vi "InitializeGUIControls.vi"(0 "Timing Plot":refnum<vi>, 1 "Save shot data":refnum<vi>, 2 "Discard shot data":refnum<vi>, 3 "Shot Quality":refnum<vi>, 4 "Fire Experiment":refnum<vi>, 5 "Abort":refnum<vi>) -> ()   [LabVIEW 2014]
doc: "Initialize various front panel GUI items. Such as reset the timing plot, disable the save/discard shot data buttons, etc."
uses:
  Controls/ShotQualityEnum.ctl
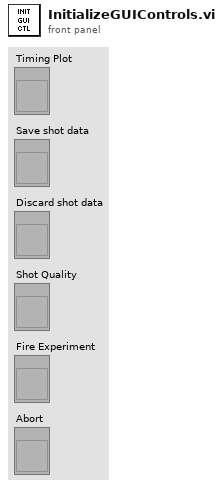
[diagram p1: front panel]
types:
  T1 = enum8{"Enabled", "Disabled", "Disabled and Grayed Out"}
  T2 = typedef "ShotQualityEnum.ctl" = enum32{"-2", "-1", "1", "2", "3", "0"}
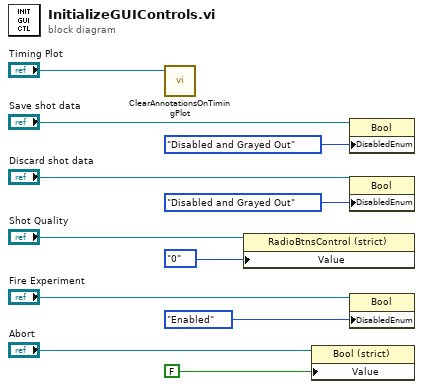
[diagram p0: block diagram]
diagram:
  n1 = call "ClearAnnotationsOnTimingPlot.vi"("Cluster in"="Timing Plot") -> ()  [unwired: 11 in]
  n2 = property class="RadioBtnsControl (strict)"(reference="Shot Quality", "Value"=ShotQualityEnum."0" ("Shot Quality")) -> ()  [unwired: 1 in, 2 out]
  n3 = property class="Bool (strict)"(reference="Abort", "Value"=FALSE) -> ()  [unwired: 1 in, 2 out]
  n4 = property class="Bool"(reference="Save shot data", "DisabledEnum"=T1."Disabled and Grayed Out" ("Disabled")) -> ()  [unwired: 1 in, 2 out]
  n5 = property class="Bool"(reference="Discard shot data", "DisabledEnum"=T1."Disabled and Grayed Out" ("Disabled")) -> ()  [unwired: 1 in, 2 out]
  n6 = property class="Bool"(reference="Fire Experiment", "DisabledEnum"=T1."Enabled" ("Disabled")) -> ()  [unwired: 1 in, 2 out]
